vi "Fill Maps.vi"(7 "Project Selected":string="DQMH Modules", 10 "Module names":string[](array[string]), 11 "DQMH Modules":refnum<vi>[](array[refnum])) -> (2 "map ref out":map{string, refnum<vi>}(c390), 3 "Tree Map out":T1)   [LabVIEW 2020, in "Panter Dashboard.lvlib"]
uses:
  Panter Dashboard.lvlib
  <vilib>/National Instruments/Tree Map/Tree Map Data.ctl
  Event types--enum.ctl
  <vilib>/National Instruments/Tree Map/Tree Map.lvlib
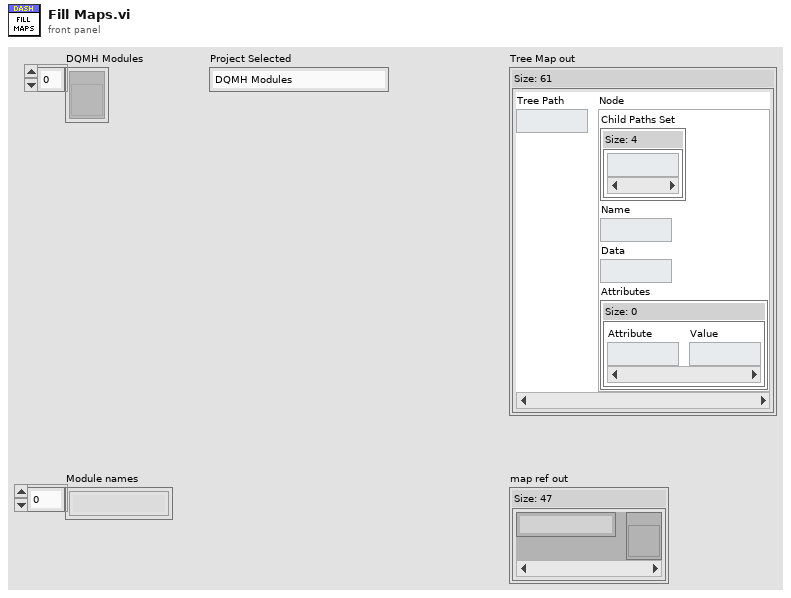
[diagram p1: front panel]
types:
  T1 = typedef "Tree Map.lvlib/Tree Map Data.ctl" = map{string, cluster{"Child Paths Set":set{string}, "Name":string, "Data":string, "Attributes":map{string, string}}}
  T2 = typedef "Panter Dashboard.lvlib/Event types--enum.ctl" = enum16{"Request", "Request and Wait for Reply", "Broadcast"}
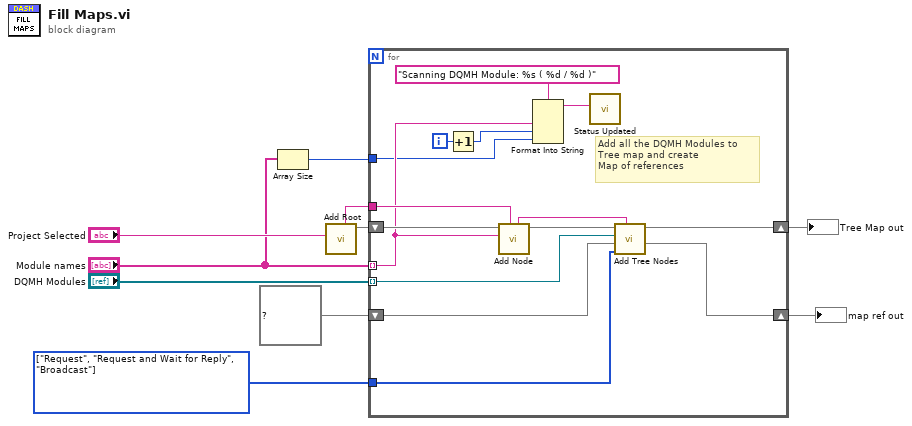
[diagram p0: block diagram]
diagram:
  w4 = T2[] [enum."Request", enum."Request and Wait for Reply", enum."Broadcast"] items=["Request", "Request and Wait for Reply", "Broadcast"] ("Event Types")
  n1 = Array Size(array="Module names") -> (size(s)=w1:i32)
  n2 = call <vilib>:"Add Root.vi"("New Root Name"="Project Selected") -> ("Tree Map Out"=w7:T1, "Root Path"=w5:string)  [unwired: 9 in]
  n3 = for {
    shift-right: [w23] -> w8
    shift-left: w7 -> [w21]
    shift-right: [w25] -> w10
    shift-left: map{string, refnum<vi>} {} ("References Map") -> [w24]
    tunnel: "DQMH Modules" -> [w17] mode=indexing
    tunnel: w5 -> [w19]
    tunnel: w4 -> [w22]
    tunnel: "Module names" -> [w16] mode=indexing
    tunnel: w1 -> [w14]
    i -> [w15]
    # "Add all the DQMH Modules to\nTree map and create \nMap of references"
    n4 = Increment(x=w15) -> (x+1=w11:i32)
    n5 = call <vilib>:"Add Node.vi"("Parent Path"=w19, "New Node Name"=w16, "Tree Map In"=w21) -> ("Tree Map Out"=w20:T1, "New Node Path"=w18:string)  [unwired: 6 in, 1 out]
    n6 = Format Into String(format string="Scanning DQMH Module: %s ( %d / %d )", w16, w11, w14) -> (resulting string=w12:string)  [unwired: 2 in, 1 out]
    n7 = call "Status Updated.vi"("Status"=w12) -> ()  [unwired: 10 in, 1 out]
    n8 = call "Add Tree Nodes.vi"("Root path"=w18, "Event Types"=w22, "map ref in"=w24, "DQMH Lib In"=w17, "Tree Map in"=w20) -> ("map ref out"=w25:map{string, refnum<vi>}, "Tree Map out"=w23:T1)  [unwired: 5 in]
  }
  "map ref out" <- w10
  "Tree Map out" <- w8
